vi "Convert CPI Module to Slot Configuration.vi"(8 "error in":errorcluster, 9 "module in":refnum<class "Module.lvclass">, 10 "RSI Module in":refnum<class "RSI Module.lvclass">, 11 "slot ref in":T1 format="%.0x") -> (0 "error out":errorcluster, 3 "slot ref out":T1 format="%.0x")   [LabVIEW 2017, in "Scan Engine Scripting.lvlib"]
uses:
  Scan Engine Scripting.lvlib
  <vilib>/NI Veristand/Custom Device API/Custom Device Item Ref.ctl
  Modules.lvlibp/RSI Module/RSI Module.lvclass
  Modules/Module/Module.lvclass
  Modules.lvlibp/SD Module/SD Module.lvclass
  C:/dev/github.com/debryant/niveristand-scan-engine-ethercat-custom-device/Custom Device Source/Modules.lvlibp/RSI Module/RSI Module.lvclass
  Modules.lvlibp/SD Module/Type Defs/Counter.ctl
  Modules.lvlibp/SD Module/Type Defs/Counter Channel.ctl
  Modules.lvlibp/SD Module/Type Defs/Count Edges.ctl
  Modules.lvlibp/SD Module/Type Defs/Period Measurement.ctl
  Modules.lvlibp/SD Module/Type Defs/Pulse Width Measurement.ctl
  Modules.lvlibp/SD Module/Type Defs/Frequency Measurement.ctl
  <vilib>/NI Veristand/Custom Device API/Custom Device API.lvlib
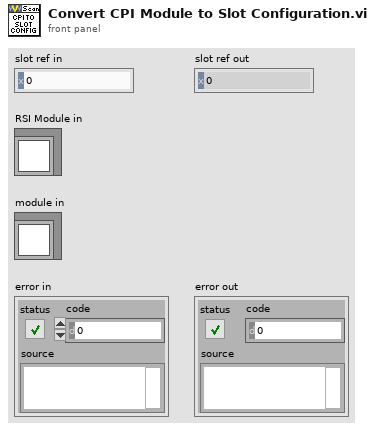
[diagram p1: front panel]
types:
  T1 = typedef "Custom Device API.lvlib/Custom Device Item Ref.ctl" = u64
  T2 = typedef "Modules.lvlibp/SD Module.lvclass/Counter Channel.ctl" = cluster{"Measurement Mode":u32, "Count Edges":T3, "Period Measurement":T4, "Pulse Width Measurement":T5, "Frequency Measurement":T6}
  T3 = typedef "Modules.lvlibp/SD Module.lvclass/Count Edges.ctl" = cluster{"Counter Event":u32, "Counter Source":u32, "Counter Direction":u32, "Terminal Count":u32, "Output Mode":u32, "Gate Mode":u32}
  T4 = typedef "Modules.lvlibp/SD Module.lvclass/Period Measurement.ctl" = cluster{"Measurement Edge":u32}
  T5 = typedef "Modules.lvlibp/SD Module.lvclass/Pulse Width Measurement.ctl" = cluster{"Measurement Type":u32}
  T6 = typedef "Modules.lvlibp/SD Module.lvclass/Frequency Measurement.ctl" = cluster{"Measurement Edge":u32, "Measurement Timebase":u32}
  T7 = typedef "Modules.lvlibp/SD Module.lvclass/Counter.ctl" = cluster{"Counter Channels":T2[]}
  T8 = typedef "Scan Engine Scripting.lvlib/counter pwm input channel settings.ctl" = cluster{"name":string, "default value":dbl, "measurement type":T9}
  T9 = typedef "Scan Engine Scripting.lvlib/PWM Input Channel.lvclass/Measurement Type.ctl" = enum16{"High Pulse", "Low Pulse", "Most Recent"}
  T10 = typedef "Modules.lvlibp/Custom Device API.lvlib/Custom Device Item Ref.ctl" = u64
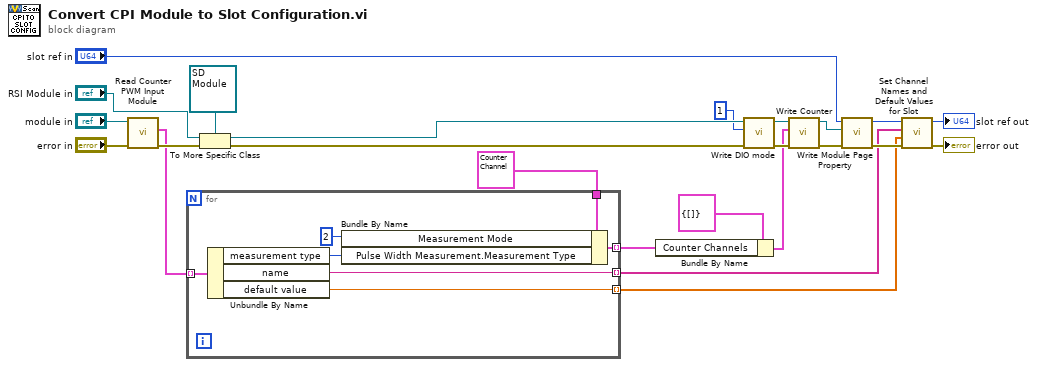
[diagram p0: block diagram]
diagram:
  n1 = call-dynamic "Read Counter PWM Input Module.vi"("error in"="error in", "module in"="module in") -> ("error out"=w15:errorcluster, "channel settings"=w3:T8[])  [unwired: 7 in, 1 out]
  n2 = for {
    tunnel: T2 {"Measurement Mode"=2, "Count Edges"={"Counter Event"=0, "Counter Source"=0, "Counter Direction"=0, "Terminal Count"=4294967295, "Output Mode"=0, "Gate Mode"=3}, "Period Measurement"={"Measurement Edge"=0}, "Pulse Width Measurement"={"Measurement Type"=3}, "Frequency Measurement"={"Measurement Edge"=0, "Measurement Timebase"=0}} ("Counter Channel") -> [w31]
    tunnel: [w30] -> w4 mode=indexing
    tunnel: w3 -> [w29] mode=indexing
    tunnel: [w26] -> w2 mode=indexing
    tunnel: [w25] -> w1 mode=indexing
    n3 = Unbundle By Name(w29) -> ("measurement type"=w28:T9, "name"=w26:string, "default value"=w25:dbl)
    n4 = Bundle By Name(cluster=w31, "Measurement Mode"=u32 2, "Pulse Width Measurement.Measurement Type"=w28) -> (w30:T2)
  }
  n5 = To More Specific Class(target class=refnum<class "SD Module.lvclass"> refnum ("Modules.lvlibp:SD Module.lvclass"), reference="RSI Module in", error in=w15) -> (specific class reference=w18:refnum<class "SD Module.lvclass">, error out=w20:errorcluster)
  n6 = Bundle By Name(cluster=T7 {"Counter Channels"=[]} ("Counter"), "Counter Channels"=w4) -> (w5:T7)
  n7 = call-dynamic "Write DIO mode.vi"("error in (no error)"=w20, "DIO mode"=u32 1, "SD Module in"=w18) -> ("error out"=w9:errorcluster, "SD Module out"=w8:refnum<class "SD Module.lvclass">)  [unwired: 7 in]
  n8 = call-dynamic "Write Counter.vi"("error in (no error)"=w9, "Counter"=w5, "SD Module in"=w8) -> ("error out"=w6:errorcluster, "SD Module out"=w7:refnum<class "SD Module.lvclass">)  [unwired: 7 in]
  n9 = call "Write Module Page Property.vi"("error in (no error)"=w6, "RSI Module"=w7, "Node Ptr In"="slot ref in") -> ("error out"=w21:errorcluster, "Node Ptr Out"=w22:T10)  [unwired: 6 in, 1 out]
  n10 = call "Set Channel Names and Default Values for Slot.vi"("error in"=w21, "default values"=w1, "channel names"=w2, "slot ref in"=w22) -> ("error out"=→"error out":errorcluster, "slot ref out"=→"slot ref out":T1)  [unwired: 6 in]
